vi "Agilent VNA Read Number of Channels Displayed.vi"(6 "Channel to be Displayed":i8=1 min=1 max=99 step=1, 7 "Agilent VNA":T1, 8 "error in (no error)":errorcluster, 11 "VISA Resource Name":refnum<visa-resource-name>) -> (0 "error out":errorcluster, 1 "Channels Displayed":i8=1 min=1 max=99 step=1, 2 "Displayed?":bool, 3 "dup VISA Resource Name":refnum<visa-resource-name>)   [LabVIEW 2011]
uses:
  TypeDefs/Agilent VNA Instrument Info.ctl
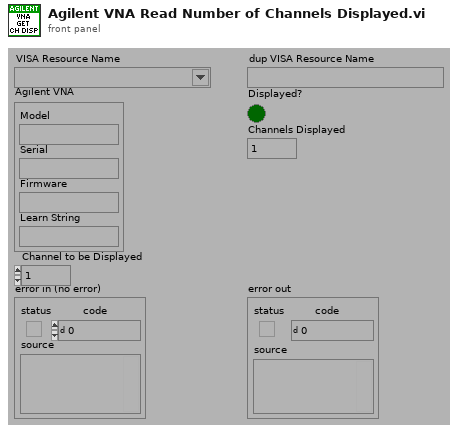
[diagram p1: front panel]
types:
  T1 = typedef "Agilent VNA Instrument Info.ctl" = cluster{"Model":string, "Serial":string, "Firmware":string, "Learn String":string}
  T2 = typedef "Agilent VNA Model.ctl" = enum16{"Not Supported", "8510X", "8719X", "8720X", "8722X", "8753X", "ENA", "PNA", "Field Fox"}
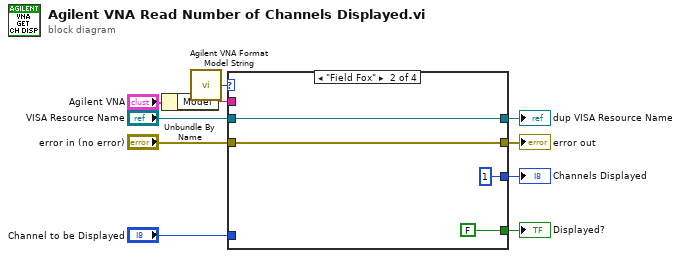
[diagram p0: block diagram]
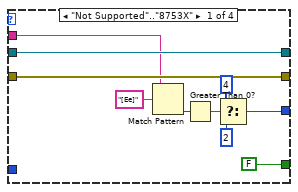
[diagram p2: hidden frame]
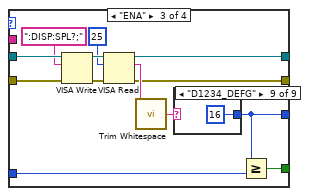
[diagram p3: hidden frame]
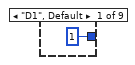
[diagram p4: hidden frame]
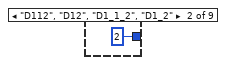
[diagram p5: hidden frame]
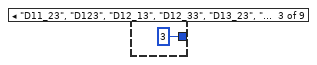
[diagram p6: hidden frame]
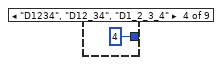
[diagram p7: hidden frame]
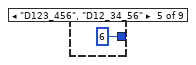
[diagram p8: hidden frame]
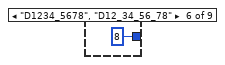
[diagram p9: hidden frame]
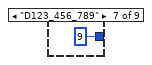
[diagram p10: hidden frame]
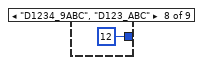
[diagram p11: hidden frame]
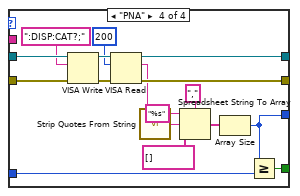
[diagram p12: hidden frame]
diagram:
  n1 = Unbundle By Name("Agilent VNA") -> ("Model"=w1:string)
  n2 = call "Agilent VNA Format Model String.vi"("Model"=w1) -> ("Model"=w10:T2)
  n3 = case shown="\"Field Fox\"" w10 {
    tunnel: "VISA Resource Name" -> [w20 w24 w37 w59]
    tunnel: "error in (no error)" -> [w19 w23 w36 w60]
    tunnel: [w20 w24 w29 w57] -> w6
    tunnel: [w19 w23 w28 w58] -> w7
    tunnel: [w12 1 ("Channels Displayed") w27 w47] -> w5
    tunnel: "Channel to be Displayed" -> [_ _ w26 w50]
    tunnel: [FALSE FALSE w25 w49] -> w3
    tunnel: w1 -> [w11 _ _ _]
    frame "Not Supported".."8753X" {
      n4 = Match Pattern(string=w11, regular expression="[Ee]") -> (offset past match=w16:i32)  [unwired: 4 out]
      n5 = Greater Than 0?(x=w16) -> (x > 0?=w15:bool)
      n6 = Select(t=i8 4 ("Channels Displayed"), s=w15, f=i8 2 ("Channels Displayed")) -> (s? t:f=w12:i8)
    }
    frame "Field Fox" {
    }
    frame "ENA" {
      n7 = VISA Write(VISA resource name=w37, write buffer=":DISP:SPL?;", error in (no error)=w36) -> (VISA resource name out=w33:refnum<visa-resource-name>, error out=w34:errorcluster)  [unwired: 1 out]
      n8 = VISA Read(VISA resource name=w33, byte count=u32 25, error in (no error)=w34) -> (VISA resource name out=w29:refnum<visa-resource-name>, read buffer=w31:string, error out=w28:errorcluster)  [unwired: 1 out]
      n9 = call <vilib>:"Trim Whitespace.vi"("string"=w31) -> ("trimmed string"=w30:string)  [unwired: 1 in]
      n10 = case shown="\"D1234_DEFG\"" w30 {
        tunnel: [i8 1 ("Channels Displayed") i8 2 ("Channels Displayed") i8 3 ("Channels Displayed") i8 4 ("Channels Displayed") i8 6 ("Channels Displayed") i8 8 ("Channels Displayed") i8 9 ("Channels Displayed") i8 12 ("Channels Displayed") i8 16 ("Channels Displayed")] -> w27
        frame "D1", Default {
        }
        frame "D112", "D12", "D1_1_2", "D1_2" {
        }
        frame "D11_23", "D123", "D12_13", "D12_33", "D13_23", "D1_2_3" {
        }
        frame "D1234", "D12_34", "D1_2_3_4" {
        }
        frame "D123_456", "D12_34_56" {
        }
        frame "D1234_5678", "D12_34_56_78" {
        }
        frame "D123_456_789" {
        }
        frame "D1234_9ABC", "D123_ABC" {
        }
        frame "D1234_DEFG" {
        }
      }
      n11 = Greater Or Equal?(x=w27, y=w26) -> (x >= y?=w25:bool)
    }
    frame "PNA" {
      n12 = VISA Write(VISA resource name=w59, write buffer=":DISP:CAT?;", error in (no error)=w60) -> (VISA resource name out=w63:refnum<visa-resource-name>, error out=w62:errorcluster)  [unwired: 1 out]
      n13 = VISA Read(VISA resource name=w63, byte count=u32 200, error in (no error)=w62) -> (VISA resource name out=w57:refnum<visa-resource-name>, read buffer=w51:string, error out=w58:errorcluster)  [unwired: 1 out]
      n14 = call "Strip Quotes From String.vi"("String In"=w51) -> ("Trimmed String"=w55:string)
      n15 = Spreadsheet String To Array(delimiter (Tab)=",", format string="%s", spreadsheet string=w55, array type (2D Dbl)=string[] []) -> (array=w48:string[])
      n16 = Array Size(array=w48) -> (size(s)=w47:i32)
      n17 = Greater Or Equal?(x=w47, y=w50) -> (x >= y?=w49:bool)
    }
  }
  "Channels Displayed" <- w5
  "dup VISA Resource Name" <- w6
  "error out" <- w7
  "Displayed?" <- w3
